vi "Obtain Blank Panel.vi"(8 "error in (no error)":errorcluster, 11 "2DArrayManager in":refnum<class "2DArrayManager.lvclass">) -> (0 "error out":errorcluster, 2 "Blank":refnum<class "2DPanelBlank.lvclass">, 3 "2DArrayManager out":refnum<class "2DArrayManager.lvclass">, 4 "Use Blank":bool)   [LabVIEW 2020, in "OOPanel.lvlib" / "2DArrayManager.lvclass"]
uses:
  2DArrayManager.lvclass
  2DArrayManager.lvclass/2DArrayManager.ctl
  Manager/Manager.lvclass
  2DPanelBlank/2DPanelBlank.lvclass
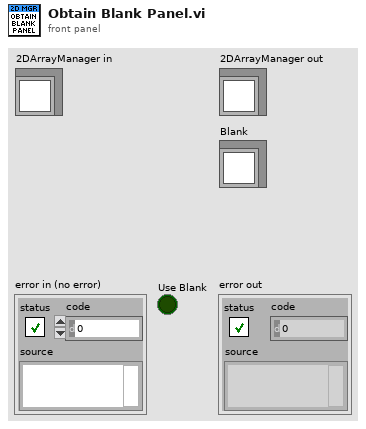
[diagram p1: front panel]
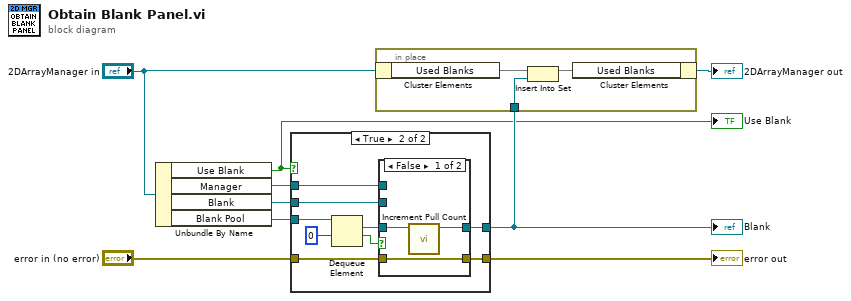
[diagram p0: block diagram]
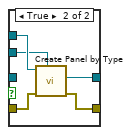
[diagram p3: hidden frame]
diagram:
  n1 = Unbundle By Name("2DArrayManager in") -> ("Use Blank"=w3:bool, "Manager"=w7:refnum<class "Manager.lvclass">, "Blank"=w8:refnum<class "2DPanelBlank.lvclass">, "Blank Pool"=w9:refnum<queue>)
  "Use Blank" <- w3
  n2 = case shown="True" w3 {
    tunnel: w9 -> [_ w19]
    tunnel: w8 -> [_ w17]
    tunnel: [_ w14] -> w5
    tunnel: w7 -> [_ w13]
    tunnel: "error in (no error)" -> [w10 w12]
    tunnel: [w10 w11] -> w1
    frame False {
    }
    frame True {
      n3 = Dequeue Element(queue=w19, timeout in ms (-1)=0) -> (element=w15:refnum<class "2DPanelBlank.lvclass">, timed out?=w16:bool)  [unwired: 1 in, 2 out]
      n4 = case shown="False" w16 {
        tunnel: w17 -> [_ w26]
        tunnel: w15 -> [w22 _]
        tunnel: [w20 w25] -> w14
        tunnel: w13 -> [_ w27]
        tunnel: w12 -> [w21 w24]
        tunnel: [w21 w23] -> w11
        frame False {
          n5 = call "Increment Pull Count.vi"("2DPanelBlank in"=w22) -> ("2DPanelBlank out"=w20:refnum<class "2DPanelBlank.lvclass">)  [unwired: 9 in, 1 out]
        }
        frame True {
          n6 = call "Create Panel by Type.vi"("Panel Type"=w26, "error in (no error)"=w24, "Manager in"=w27) -> ("error out"=w23:errorcluster, "Panel"=w25:refnum<class "2DPanelBlank.lvclass">)  [unwired: 6 in, 1 out]
        }
      }
    }
  }
  "error out" <- w1
  "Blank" <- w5
  n7 = in-place {
    in-place-border: w5 -> [w28]
    n8 = in-place-cluster #1("2DArrayManager in") -> ("Used Blanks"=w30:set{refnum<class "2DPanelBlank.lvclass">})
    n9 = Insert Into Set(10:w28, 11:w30) -> (3:w29:set{refnum<class "2DPanelBlank.lvclass">})  [unwired: 1 out]
    n10 = in-place-cluster #1("Used Blanks"=w29) -> (→"2DArrayManager out":refnum<class "2DArrayManager.lvclass">)
  }
